vi "constant--blank_chess_square.vi"() -> (0 "blank_chess_square":T1)   [LabVIEW 2020, in "core.lvlib" / "core_data.lvlib"]
uses:
  core_data.lvlib
  chess_square.ctl
  neighbour_square.ctl
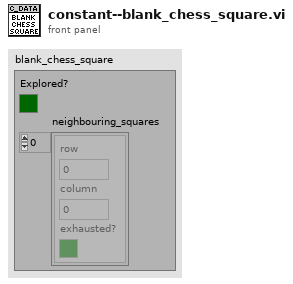
[diagram p1: front panel]
types:
  T1 = typedef "core.lvlib/core_data.lvlib/chess_square.ctl" = cluster{"Explored?":bool, "neighbouring_squares":T2[]}
  T2 = typedef "core.lvlib/core_data.lvlib/neighbour_square.ctl" = cluster{"row":u8, "column":u8, "exhausted?":bool}
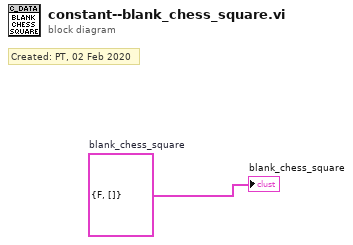
[diagram p0: block diagram]
diagram:
  w1 = T1 {"Explored?"=FALSE, "neighbouring_squares"=[]}  # blank_chess_square
  # "Created: PT, 02 Feb 2020"
  "blank_chess_square" <- w1
